vi "End Program.vi"(8 "error in (no error)":errorcluster, 11 "controller":refnum<k24>) -> (0 "error out":errorcluster)   [LabVIEW 2011]
uses:
  C:/Users/Admin/Desktop/Gantry Code Transfer/source/Code Transfer/Aerotech.A3200.dll
  Aerotech.A3200.dll
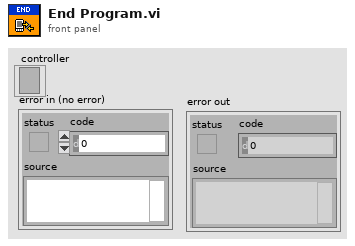
[diagram p1: front panel]
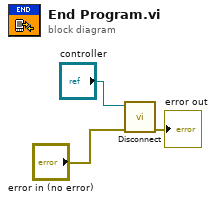
[diagram p0: block diagram]
diagram:
  n1 = call "Disconnect.vi"("error in (no error)"="error in (no error)", "controller"="controller") -> ("error out"=→"error out":errorcluster)  [unwired: 9 in]
